vi "Create Task Wrapper.vi"(0 "Task map in":map{string, refnum<k21>}(c390), 5 "Message Data in":T3, 11 "error in (no error)":errorcluster) -> (4 "Task map out":map{string, refnum<k21>}(c390), 6 "Message Data out":T1, 15 "error out":errorcluster)   [LabVIEW 2021, in "NI DAQmx_wrapper.lvlib"]
uses:
  NI DAQmx_wrapper.lvlib
  NI DAQmx_server/RPC Messages/nidevice_grpc_SessionInitializationBehavior.ctl
  NI DAQmx_server/NI DAQmx_server.lvlib
  NI DAQmx_server/RPC Messages/nidaqmx_grpc_CreateTaskRequest.ctl
  NI DAQmx_server/RPC Messages/nidevice_grpc_Session_session/nidevice_grpc_Session_session.lvclass
  NI DAQmx_server/RPC Messages/nidevice_grpc_Session.ctl
  NI DAQmx_server/RPC Messages/nidaqmx_grpc_CreateTaskResponse.ctl
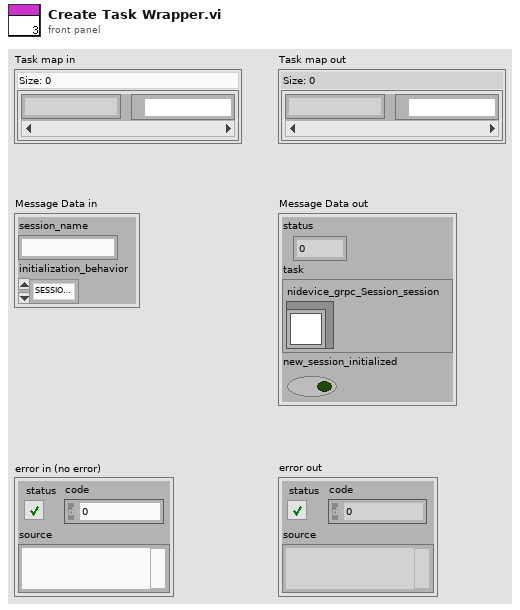
[diagram p1: front panel]
types:
  T1 = typedef "NI DAQmx_server.lvlib/nidaqmx_grpc_CreateTaskResponse.ctl" = cluster{"status":i32, "task":T2, "new_session_initialized":bool}
  T2 = typedef "NI DAQmx_server.lvlib/nidevice_grpc_Session.ctl" = cluster{"nidevice_grpc_Session_session":refnum<class "nidevice_grpc_Session_session.lvclass">}
  T3 = typedef "NI DAQmx_server.lvlib/nidaqmx_grpc_CreateTaskRequest.ctl" = cluster{"session_name":string, "initialization_behavior":T4}
  T4 = typedef "NI DAQmx_server.lvlib/nidevice_grpc_SessionInitializationBehavior.ctl" = enum32{"SESSION_INITIALIZATION_BEHAVIOR_UNSPECIFIED", "SESSION_INITIALIZATION_BEHAVIOR_INITIALIZE_NEW", "SESSION_INITIALIZATION_BEHAVIOR_ATTACH_TO_EXISTING"}
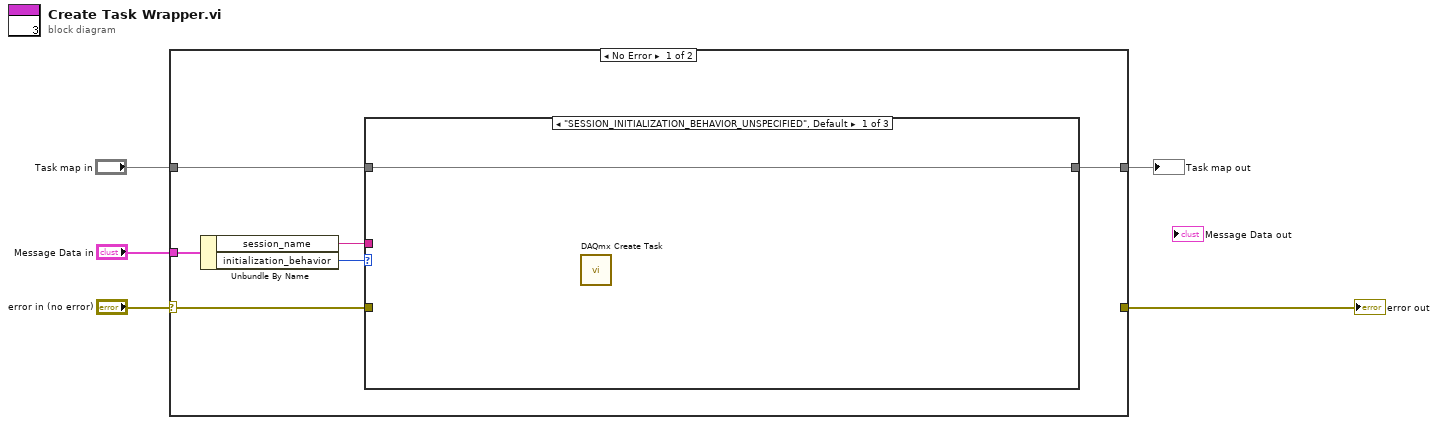
[diagram p0: block diagram]
diagram:
  n1 = case shown="No Error" "error in (no error)" {
    selector: "error in (no error)" -> [w8 w13]
    tunnel: [_ w13] -> w4
    tunnel: "Message Data in" -> [w11 _]
    tunnel: "Task map in" -> [w9 _]
    tunnel: [w6 _] -> w1
    frame No Error {
      n2 = Unbundle By Name(w11) -> ("session_name"=w7:string, "initialization_behavior"=w10:T4)
      n3 = case shown="\"SESSION_INITIALIZATION_BEHAVIOR_UNSPECIFIED\", Default" w10 {
        tunnel: w9 -> [w12 _ _]
        tunnel: w8 -> [_ _ _]
        tunnel: w7 -> [_ _ _]
        tunnel: [w12 _ _] -> w6
        frame "SESSION_INITIALIZATION_BEHAVIOR_UNSPECIFIED", Default {
          n4 = call <vilib>:"DAQmx Create Task.vi"() -> ()  [unwired: 14 in, 2 out]
        }
        frame "SESSION_INITIALIZATION_BEHAVIOR_INITIALIZE_NEW" {
        }
        frame "SESSION_INITIALIZATION_BEHAVIOR_ATTACH_TO_EXISTING" {
        }
      }
    }
    frame Error {
    }
  }
  "error out" <- w4
  "Task map out" <- w1
